vi "To Variant.vi"(8 "error in":errorcluster, 9 "type code":T1, 10 "default":variant, 11 "Value in":refnum<class "Value.lvclass">) -> (0 "error out":errorcluster, 2 "value":variant, 3 "Value out":refnum<class "Value.lvclass">, 5 "timestamp":timestamp)   [LabVIEW 2020, in "Value.lvlib" / "Value.lvclass"]
uses:
  Value.lvclass
  Value.lvclass/Value.ctl
  Type Code.ctl
  Value.lvlib
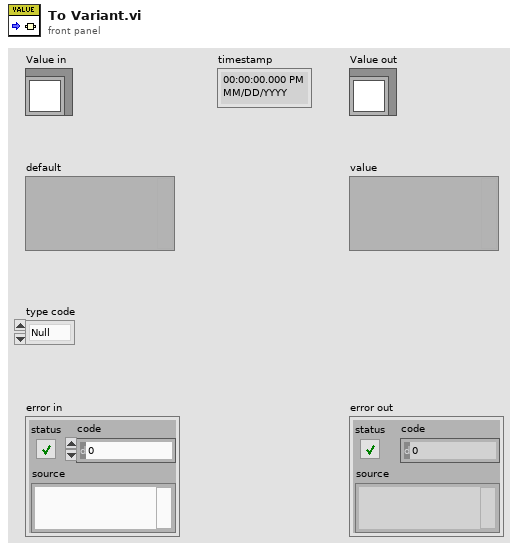
[diagram p1: front panel]
types:
  T1 = typedef "Value.lvlib/Type Code.ctl" = enum8{"Null", "Bool", "BoolA", "Int8", "Int8A", "Int16", "Int16A", "Int32", "Int32A", "Int64", "Int64A", "UInt8", "UInt8A", "UInt16", "UInt16A", "UInt32", "UInt32A", "UInt64", "UInt64A", "Float32", "Float32A", "Float64", "Float64A", "String", "StringA", "Struct", "StructA", "Union", "UnionA", "Any", "AnyA"}
  T2 = typedef "Value.lvlib/Display Metadata.ctl" = cluster{"Limit Low":dbl, "Limit High":dbl, "Description":string, "Units":string, "Precision":i32, "Form":enum32{"Default", "String", "Binary", "Decimal", "Hex", "Exponential", "Engineering"}}
  T3 = typedef "Value.lvlib/Control Metadata.ctl" = cluster{"Limit Low":dbl, "Limit High":dbl, "Min Step":dbl}
  T4 = typedef "Value.lvlib/Alarm Status.ctl" = cluster{"Severity":T5, "Status":enum32{"no", "device", "driver", "record", "db", "conf", "undefined", "client"}, "Message":string}
  T5 = typedef "Value.lvlib/Alarm Severity.ctl" = enum32{"no", "minor", "major", "record", "invalid", "undefined", ""}
  T6 = typedef "Value.lvlib/Alarm Limits.ctl" = cluster{"Active":bool, "Low Alarm Limit":dbl, "Low Warning Limit":dbl, "High Warning Limit":dbl, "High Alarm Limit":dbl, "Low Alarm Severity":T5, "Low Warning Severity":T5, "High Warning Severity ":T5, "High Alarm Severity":T5, "Hysteresis":dbl}
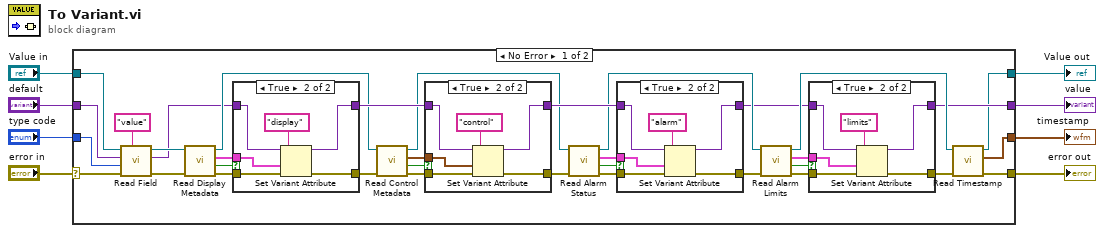
[diagram p0: block diagram]
diagram:
  n1 = case shown="No Error" "error in" {
    selector: "error in" -> [w16 w77]
    tunnel: "Value in" -> [w12 w76]
    tunnel: [w40 w77] -> w5
    tunnel: [w20 _] -> w4
    tunnel: [w18 _] -> w6
    tunnel: [w17 w76] -> w3
    tunnel: "default" -> [w10 _]
    tunnel: "type code" -> [w9 _]
    frame No Error {
      n2 = call "Read Field.vi"("field name"="value", "error in (no error)"=w16, "type code"=w9, "value"=w10, "Value in"=w12) -> ("error out"=w15:errorcluster, "value out"=w13:variant, "Value out"=w14:refnum<class "Value.lvclass">)  [unwired: 4 in]
      n3 = call "Read Display Metadata.vi"("error in"=w15, "Value in"=w14) -> ("error out"=w42:errorcluster, "has display metadata?"=w43:bool, "display metadata"=w41:T2, "Value out"=w30:refnum<class "Value.lvclass">)  [unwired: 6 in]
      n4 = case shown="True" w43 {
        tunnel: w42 -> [w69 w75]
        tunnel: [w69 w74] -> w35
        tunnel: w41 -> [_ w73]
        tunnel: w13 -> [w68 w72]
        tunnel: [w68 w70] -> w32
        frame False {
        }
        frame True {
          n5 = Set Variant Attribute(Variant=w72, name="display", value=w73, error in=w75) -> (Variant out=w70:variant, error out=w74:errorcluster)  [unwired: 1 out]
        }
      }
      n6 = call "Read Control Metadata.vi"("error in"=w35, "Value in"=w30) -> ("error out"=w33:errorcluster, "has control metadata?"=w34:bool, "control metadata"=w28:T3, "Value out"=w29:refnum<class "Value.lvclass">)  [unwired: 6 in]
      n7 = case shown="True" w34 {
        tunnel: w33 -> [w53 w59]
        tunnel: [w53 w58] -> w36
        tunnel: w28 -> [_ w57]
        tunnel: w32 -> [w52 w56]
        tunnel: [w52 w54] -> w31
        frame False {
        }
        frame True {
          n8 = Set Variant Attribute(Variant=w56, name="control", value=w57, error in=w59) -> (Variant out=w54:variant, error out=w58:errorcluster)  [unwired: 1 out]
        }
      }
      n9 = call "Read Alarm Status.vi"("error in"=w36, "Value in"=w29) -> ("error out"=w39:errorcluster, "has alarm status?"=w37:bool, "alarm status"=w38:T4, "Value out"=w23:refnum<class "Value.lvclass">)  [unwired: 6 in]
      n10 = case shown="True" w37 {
        tunnel: w39 -> [w61 w67]
        tunnel: [w61 w66] -> w27
        tunnel: w38 -> [_ w65]
        tunnel: w31 -> [w60 w62]
        tunnel: [w60 w63] -> w21
        frame False {
        }
        frame True {
          n11 = Set Variant Attribute(Variant=w62, name="alarm", value=w65, error in=w67) -> (Variant out=w63:variant, error out=w66:errorcluster)  [unwired: 1 out]
        }
      }
      n12 = call "Read Alarm Limits.vi"("error in"=w27, "Value in"=w23) -> ("error out"=w26:errorcluster, "has alarm limits?"=w25:bool, "alarm limits"=w24:T6, "Value out"=w22:refnum<class "Value.lvclass">)  [unwired: 6 in]
      n13 = case shown="True" w25 {
        tunnel: w26 -> [w45 w51]
        tunnel: [w45 w50] -> w19
        tunnel: w24 -> [_ w49]
        tunnel: w21 -> [w44 w46]
        tunnel: [w44 w47] -> w20
        frame False {
        }
        frame True {
          n14 = Set Variant Attribute(Variant=w46, name="limits", value=w49, error in=w51) -> (Variant out=w47:variant, error out=w50:errorcluster)  [unwired: 1 out]
        }
      }
      n15 = call "Read Timestamp.vi"("error in"=w19, "Value in"=w22) -> ("error out"=w40:errorcluster, "timestamp"=w18:timestamp, "Value out"=w17:refnum<class "Value.lvclass">)  [unwired: 7 in]
    }
    frame Error {
    }
  }
  "timestamp" <- w6
  "error out" <- w5
  "value" <- w4
  "Value out" <- w3
